vi "Low Pass Differentiator Test.vi"() -> ()   [LabVIEW 2011]
doc: "Tests the low-pass differentiator by inputting a triangle wave, with the optional addition of random noise. Visually displays output."
panel:
  out "Array":dbl[](array[numeric])
  in  "Intermittent\nData":bool=TRUE
  in  "Random\nNoise":bool=TRUE
  in  "Smoothing Factor":dbl=0.1
  in  "slew rate":dbl=1.0
  out "Waveform Chart":cluster{dbl, "dX, smoothed":dbl}(graph)
  in  "stop":bool
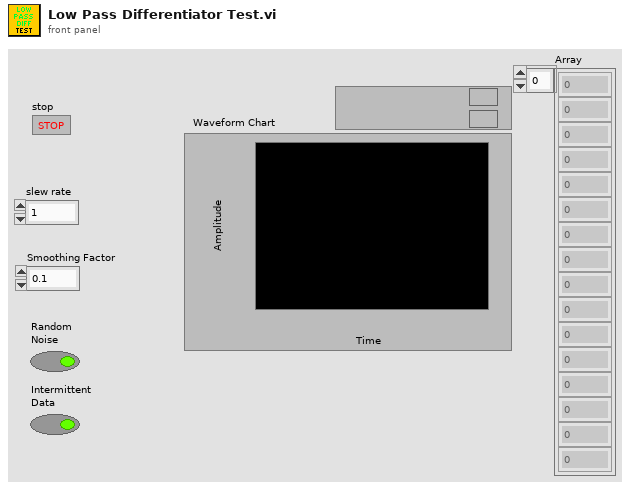
[diagram p1: front panel]
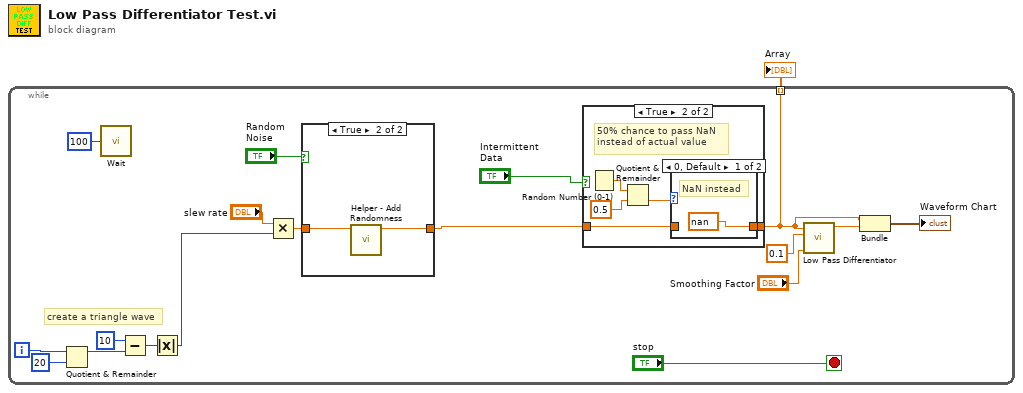
[diagram p0: block diagram]
diagram:
  n1 = while {
    tunnel: [w2] -> w1 mode=indexing
    i -> [w18]
    stop <- "stop" stop-if-true
    # "create a triangle wave"
    n2 = Quotient & Remainder(x=w18, y=20) -> (x-y*floor(x/y)=w16:i32)  [unwired: 1 out]
    n3 = call "Wait"("Count(mSec)"=u32 100) -> ()  [unwired: 1 out]
    n4 = Subtract(x=10 ("y"), y=w16) -> (x-y=w14:i32)
    n5 = Absolute Value(x=w14) -> (abs(x)=w12:i32)
    n6 = Multiply(x="slew rate", y=w12) -> (x*y=w6:dbl)
    n7 = case shown="True" "Random\nNoise" {
      tunnel: [w28 w30] -> w4
      tunnel: w6 -> [w28 w29]
      frame False {
      }
      frame True {
        n8 = call "Helper - Add Randomness.vi"("Numeric in"=w29) -> ("Numeric out"=w30:dbl)  [unwired: 10 in]
      }
    }
    n9 = case shown="True" "Intermittent\nData" {
      tunnel: [w20 w22] -> w2
      tunnel: w4 -> [w20 w21]
      frame False {
      }
      frame True {
        # "50% chance to pass NaN\ninstead of actual value"
        n10 = Random Number (0-1)() -> (number: 0 to 1=w25:dbl)
        n11 = Quotient & Remainder(x=w25, y=0.5) -> (floor(x/y)=w23:dbl)  [unwired: 1 out]
        n12 = case shown="0, Default" w23 {
          tunnel: [nan w27] -> w22
          tunnel: w21 -> [_ w27]
          frame 0, Default {
            # "NaN instead"
          }
          frame 1 {
            # "go on\nthrough"
          }
        }
      }
    }
    n13 = call "Low Pass Differentiator.vi"("Smoothing Factor"="Smoothing Factor", "dt"=0.1, "X"=w2) -> ("dX, smoothed"=w10:dbl)  [unwired: 8 in]
    n14 = Bundle("Numeric out"=w2, "dX, smoothed"=w10) -> (→"Waveform Chart":cluster{"Numeric out":dbl, "dX, smoothed":dbl})  [unwired: 1 in]
  }
  "Array" <- w1
